vi "Close.vi"(8 "error in":errorcluster, 11 "Gradient in":refnum<class "Gradient.lvclass">) -> (0 "error out":errorcluster, 3 "Gradient out":refnum<class "Gradient.lvclass">)   [LabVIEW 2023, in "Gradient.lvclass"]
uses:
  Gradient.lvclass
  <vilib>/ADAS Replay HIL/AdasHilServices/AdasHilChannelServices.lvlib
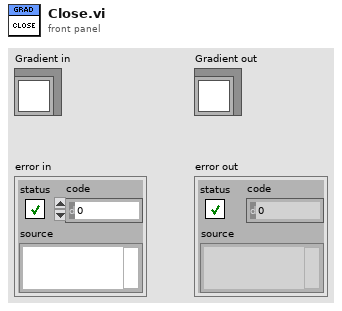
[diagram p1: front panel]
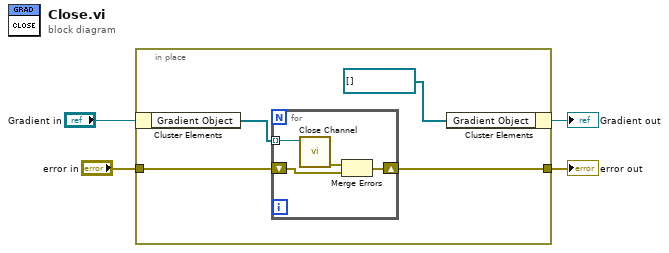
[diagram p0: block diagram]
diagram:
  n1 = in-place {
    in-place-border: [w8] -> w1
    in-place-border: "error in" -> [w5]
    n2 = in-place-cluster #1("Gradient in") -> ("Gradient Object"=w7:refnum<k21>[])
    n3 = for {
      tunnel: w7 -> [w12] mode=indexing
      shift-right: [w9] -> w8
      shift-left: w5 -> [w10]
      n4 = call <vilib>:"Close Channel.vi"("ADAS HIL Channel"=w12) -> ("error out"=w11:errorcluster)  [unwired: 10 in]
      n5 = Merge Errors(w11, w10) -> (w9:errorcluster)
    }
    n6 = in-place-cluster #1("Gradient Object"=refnum<k21>[] [] ("Actual Value Object")) -> (→"Gradient out":refnum<class "Gradient.lvclass">)
  }
  "error out" <- w1
